vi "1C.1 SmallRCSense.vi"(10 "Wind Direction":T3=45.0 format="%05.1f", 11 "Wind Speed":dbl=1.0) -> (0 "Apparent Wind\nSpeed":T1, 1 "Apparent Wind\nDirection":T2, 2 "Boat\nVelocity":T4, 3 "Heading":T3 format="%05.1f", 4 "Eye in the Sky":T6(plugin-control), 5 "Boat Location":T5)   [LabVIEW 2011]
doc: "TODO: finish camera interpreter\nTODO: arrange this to be easier to convert for future boats!"
uses:
  2-RIO/2 Typedefs/UTM Location.ctl
  2-RIO/2 Typedefs/Velocity.ctl
  2-RIO/2 Typedefs/heading.ctl
  2-RIO/2 Typedefs/apparent wind direction.ctl
  2-RIO/2 Typedefs/apparent wind speed.ctl
  2-RIO/2 Globals/2 Global.vi
panel:
  out "Frame Rate (Hz)":dbl
  out "Apparent Wind\nin global ref frame":T4
  out "Absolute Wind":T4
  in  "Add Randomness\nTo Wind Measurement":bool
  # "TODO: upgrade speed + reliability of pattern matching"
  # "(in boat ref frame)"
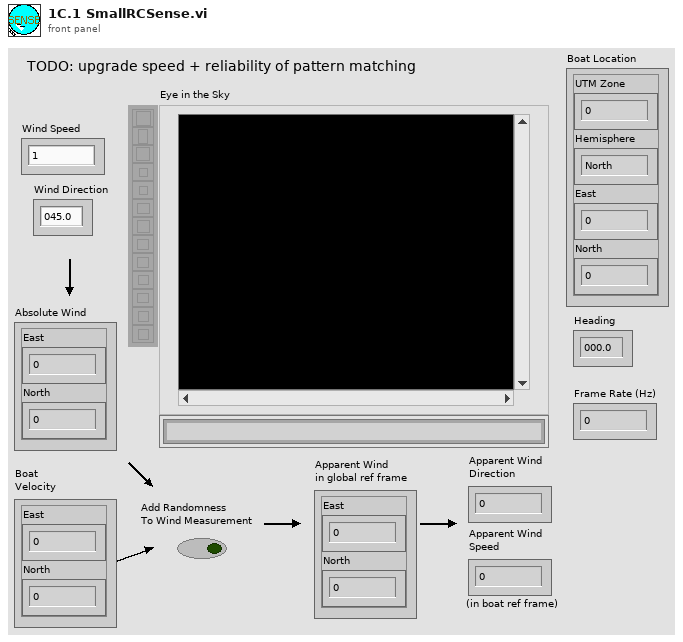
[diagram p1: front panel]
types:
  T1 = typedef "apparent wind speed.ctl" = dbl
  T2 = typedef "apparent wind direction.ctl" = dbl
  T3 = typedef "heading.ctl" = dbl
  T4 = typedef "Velocity.ctl" = cluster{"East":dbl, "North":dbl}
  T5 = typedef "UTM Location.ctl" = cluster{"UTM Zone":dbl, "Hemisphere":enum16{"North", "South"}, "East":dbl, "North":dbl}
  T6 = typedef "IMAQ Image.ctl" = refnum<image>
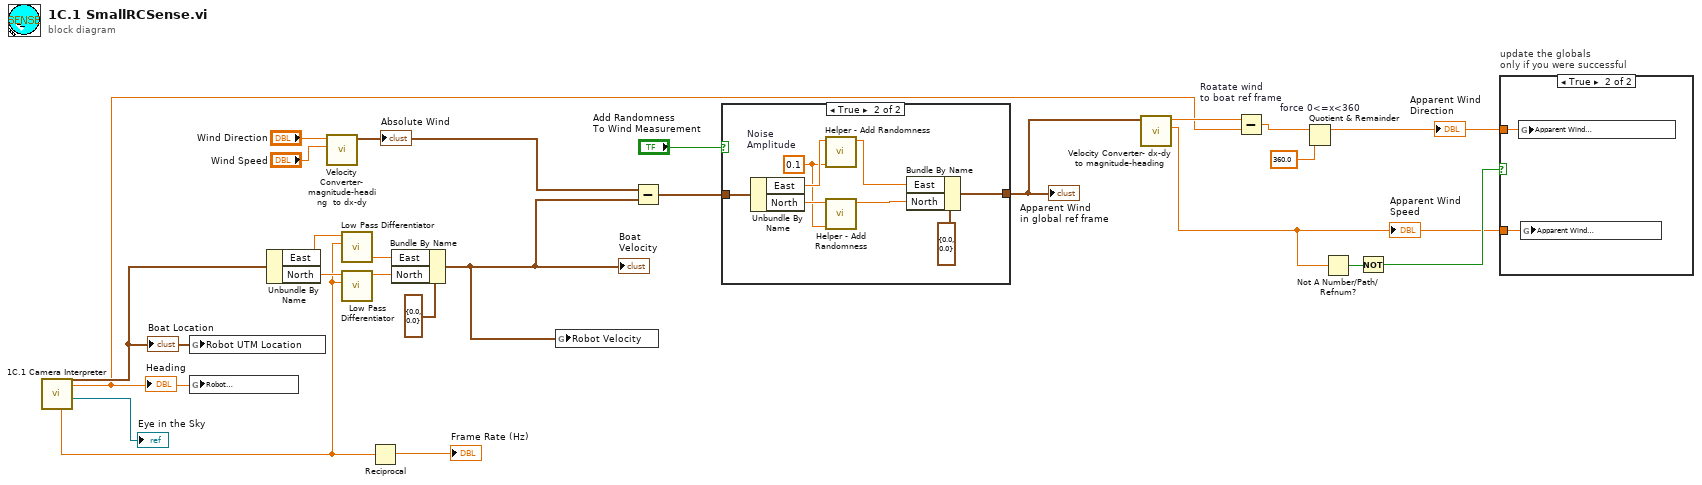
[diagram p0: block diagram]
diagram:
  n1 = call "1C.1 Camera Interpreter.vi"() -> ("Overhead Image"=→"Eye in the Sky":T6, "Heading"=w6:T3, "Boat Location"=w7:T5, "Time Elapsed (s)\nSince Last Image"=w12:dbl)  [unwired: 7 in, 1 out]
  "Boat Location" <- w7
  "Heading" <- w6
  n2 = global write "2 Global.vi" "Robot UTM Location"(w7) -> ()
  n3 = global write "2 Global.vi" "Robot\nHeading"(w6) -> ()
  n4 = Unbundle By Name(w7) -> ("East"=w23:dbl, "North"=w22:dbl)
  n5 = call "Velocity Converter- magnitude-heading  to dx-dy.vi"("Magnitude"="Wind Speed", "Heading"="Wind Direction") -> ("Vector Out"=w15:T4)  [unwired: 9 in]
  "Absolute Wind" <- w15
  n6 = call "Low Pass Differentiator.vi"("dt"=w12, "X"=w23) -> ("dX, smoothed"=w20:dbl)  [unwired: 9 in]
  n7 = call "Low Pass Differentiator.vi"("dt"=w12, "X"=w22) -> ("dX, smoothed"=w21:dbl)  [unwired: 9 in]
  n8 = Reciprocal(x=w12) -> (1/x=→"Frame Rate (Hz)":dbl)
  n9 = Bundle By Name(cluster=T4 {"East"=0.0, "North"=0.0} ("Velocity 2"), "East"=w20, "North"=w21) -> (w2:T4)
  "Boat\nVelocity" <- w2
  n10 = global write "2 Global.vi" "Robot Velocity"(w2) -> ()
  n11 = Subtract(x=w15, y=w2) -> (x-y=w19:T4)
  n12 = case shown="True" "Add Randomness\nTo Wind Measurement" {
    tunnel: [w25 w33] -> w9
    tunnel: w19 -> [w25 w32]
    frame False {
    }
    frame True {
      w27 = 0.1  # Noise Amplitude
      n13 = Unbundle By Name(w32) -> ("East"=w31:dbl, "North"=w30:dbl)
      n14 = call "Helper - Add Randomness.vi"("Amplitude\n(default 1)"=w27, "Numeric in"=w31) -> ("Numeric out"=w28:dbl)  [unwired: 9 in]
      n15 = call "Helper - Add Randomness.vi"("Amplitude\n(default 1)"=w27, "Numeric in"=w30) -> ("Numeric out"=w29:dbl)  [unwired: 9 in]
      n16 = Bundle By Name(cluster=T4 {"East"=0.0, "North"=0.0} ("Apparent Wind 2"), "East"=w28, "North"=w29) -> (w33:T4)
    }
  }
  "Apparent Wind\nin global ref frame" <- w9
  n17 = call "Velocity Converter- dx-dy to magnitude-heading.vi"("Vector In"=w9) -> ("Magnitude Out"=w3:dbl, "Heading Out"=w11:T3)  [unwired: 9 in]
  "Apparent Wind\nSpeed" <- w3
  n18 = Subtract "Roatate wind\nto boat ref frame"(x=w11, y=w6) -> (x-y=w1:T3)
  n19 = Quotient & Remainder "force 0<=x<360"(x=w1, y=T3 360.0) -> (x-y*floor(x/y)=w8:T3)  [unwired: 1 out]
  "Apparent Wind\nDirection" <- w8
  n20 = Not A Number/Path/Refnum?(number/path/refnum=w3) -> (NaN/Path/Refnum?=w5:bool)
  n21 = Not(x=w5) -> (.not. x?=w4:bool)
  n22 = case "update the globals\nonly if you were successful" shown="True" w4 {
    tunnel: w8 -> [_ w35]
    tunnel: w3 -> [_ w34]
    frame False {
    }
    frame True {
      n23 = global write "2 Global.vi" "Apparent Wind\nDirection"(w35) -> ()
      n24 = global write "2 Global.vi" "Apparent Wind\nSpeed"(w34) -> ()
    }
  }
